vi "Test_I2C_eeprom_read.vi"(6 "VISA resource name":refnum<visa-resource-name>, 7 "Passed so far?":bool, 8 "error in (no error)":errorcluster, 11 "Slot":T1) -> (0 "error out":errorcluster, 3 "Product ID":string, 4 "VISA resource name out":refnum<visa-resource-name>, 5 "Passed?":bool)   [LabVIEW 2024]
uses:
  AP slots to test.ctl
panel:
  out "read buffer":string
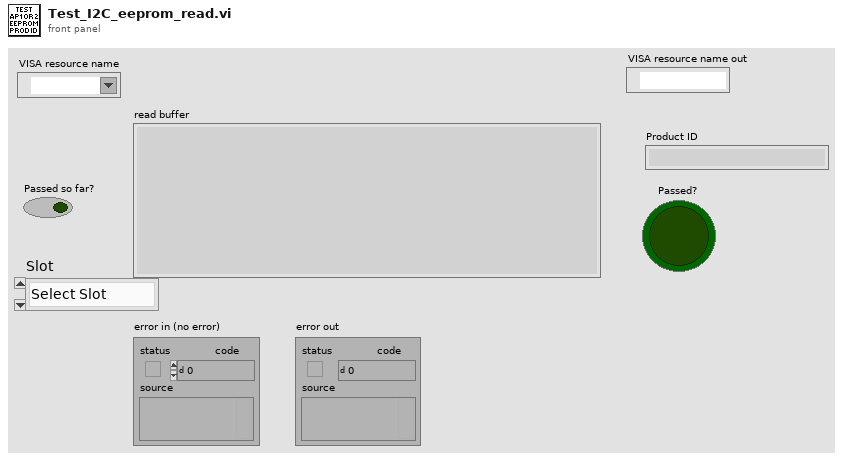
[diagram p1: front panel]
types:
  T1 = typedef "AP slots to test.ctl" = enum16{"Select Slot", "AP1", "AP2", "AP1 and AP2"}
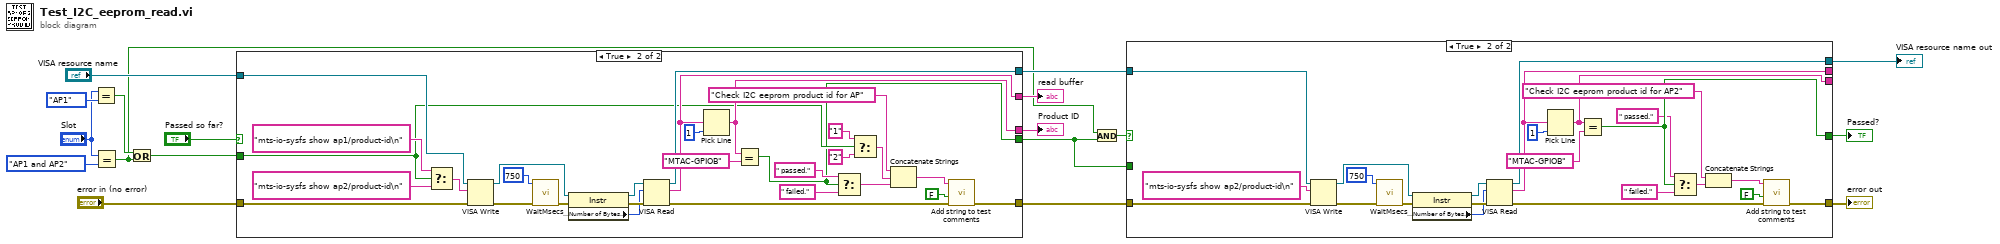
[diagram p0: block diagram]
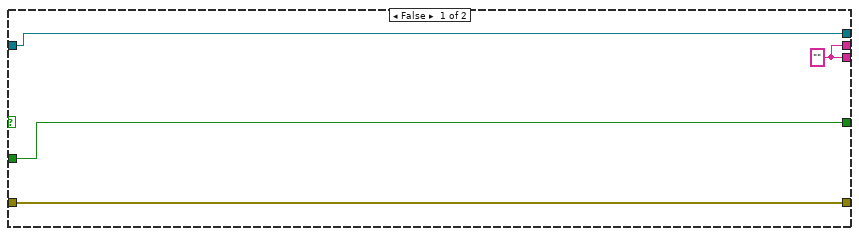
[diagram p2: hidden frame]
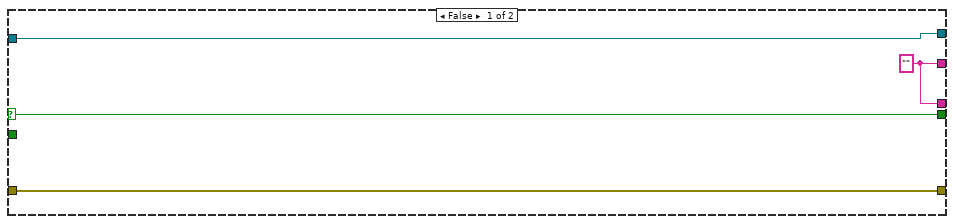
[diagram p3: hidden frame]
diagram:
  n1 = Equal?(x="Slot", y=AP_slots_to_test."AP1") -> (x = y?=w11:bool)
  n2 = Equal?(x="Slot", y=AP_slots_to_test."AP1 and AP2") -> (x = y?=w3:bool)
  n3 = Or(x=w11, y=w3) -> (x .or. y?=w12:bool)
  n4 = case shown="True" "Passed so far?" {
    selector: "Passed so far?" -> [w21 _]
    tunnel: [w22 w25] -> w7
    tunnel: w12 -> [_ w33]
    tunnel: [w21 w23] -> w1
    tunnel: "VISA resource name" -> [w20 w40]
    tunnel: [w19 w39] -> w17
    tunnel: [w19 w38] -> w14
    tunnel: "error in (no error)" -> [w22 w37]
    tunnel: [w20 w36] -> w8
    frame False {
      w19 = "" ("output string")
    }
    frame True {
      n5 = Select(t="mts-io-sysfs show ap1/product-id\n", s=w33, f="mts-io-sysfs show ap2/product-id\n") -> (s? t:f=w44:string)
      n6 = VISA Write(VISA resource name=w40, write buffer=w44, error in (no error)=w37) -> (VISA resource name out=w42:refnum<visa-resource-name>, error out=w43:errorcluster)  [unwired: 1 out]
      n7 = call "WaitMsecs.vi"("error in (no error)"=w43, "Wait Msecs"=u32 750) -> ("error out"=w45:errorcluster)  [unwired: 9 in]
      n8 = property class="Instr"(reference=w42, error in=w45) -> (reference out=w52:refnum<visa-resource-name>, error out=w51:errorcluster, "Serial Settings:Number of Bytes at Serial Port"=w50:u32)
      n9 = VISA Read(VISA resource name=w52, byte count=w50, error in (no error)=w51) -> (VISA resource name out=w36:refnum<visa-resource-name>, read buffer=w38:string, error out=w35:errorcluster)  [unwired: 1 out]
      n10 = Pick Line(multi-line string=w38, line index=1) -> (output string=w39:string)  [unwired: 1 in]
      n11 = Equal?(x=w39, y="MTAC-GPIOB") -> (x = y?=w23:bool)
      n12 = Select(t=" passed.", s=w23, f=" failed.") -> (s? t:f=w27:string)
      n13 = Select(t="1", s=w33, f="2") -> (s? t:f=w30:string)
      n14 = Concatenate Strings("Check I2C eeprom product id for AP" ("string"), w30, w27) -> (w26:string)
      n15 = call "Add string to test comments.vi"("error in (no error)"=w35, "New Section (y)?"=FALSE, "Comments"=w26) -> ("error out"=w25:errorcluster)  [unwired: 7 in, 1 out]
    }
  }
  "Product ID" <- w17
  "read buffer" <- w14
  n16 = And(x=w3, y=w1) -> (x .and. y?=w2:bool)
  n17 = case shown="True" w2 {
    tunnel: [w56 w59] -> w6
    tunnel: [w53 w64] -> w5
    tunnel: w8 -> [w55 w71]
    tunnel: [w54 w70] -> _
    tunnel: [w54 w69] -> _
    tunnel: w7 -> [w56 w68]
    tunnel: [w55 w67] -> w4
    tunnel: w1 -> [w53 _]
    frame False {
      w54 = "" ("output string")
    }
    frame True {
      n18 = VISA Write(VISA resource name=w71, write buffer="mts-io-sysfs show ap2/product-id\n", error in (no error)=w68) -> (VISA resource name out=w73:refnum<visa-resource-name>, error out=w74:errorcluster)  [unwired: 1 out]
      n19 = call "WaitMsecs.vi"("error in (no error)"=w74, "Wait Msecs"=u32 750) -> ("error out"=w75:errorcluster)  [unwired: 9 in]
      n20 = property class="Instr"(reference=w73, error in=w75) -> (reference out=w80:refnum<visa-resource-name>, error out=w79:errorcluster, "Serial Settings:Number of Bytes at Serial Port"=w78:u32)
      n21 = VISA Read(VISA resource name=w80, byte count=w78, error in (no error)=w79) -> (VISA resource name out=w67:refnum<visa-resource-name>, read buffer=w69:string, error out=w66:errorcluster)  [unwired: 1 out]
      n22 = Pick Line(multi-line string=w69, line index=1) -> (output string=w70:string)  [unwired: 1 in]
      n23 = Equal?(x=w70, y="MTAC-GPIOB") -> (x = y?=w64:bool)
      n24 = Select(t=" passed.", s=w64, f=" failed.") -> (s? t:f=w61:string)
      n25 = Concatenate Strings("Check I2C eeprom product id for AP2" ("string"), w61) -> (w60:string)
      n26 = call "Add string to test comments.vi"("error in (no error)"=w66, "New Section (y)?"=FALSE, "Comments"=w60) -> ("error out"=w59:errorcluster)  [unwired: 7 in, 1 out]
    }
  }
  "error out" <- w6
  "Passed?" <- w5
  "VISA resource name out" <- w4
